vi "ClearTable.vi"(8 "error in":errorcluster, 10 "Table Name":string, 11 "Path":path) -> (0 "error out":errorcluster, 1 "OK？":bool, 2 "Table Name":string, 3 "Path":path)   [LabVIEW 2017, in "SQLite.lvlib"]
uses:
  SQLite.lvlib
  Core/Tables/SQLite_Clear Table.vi
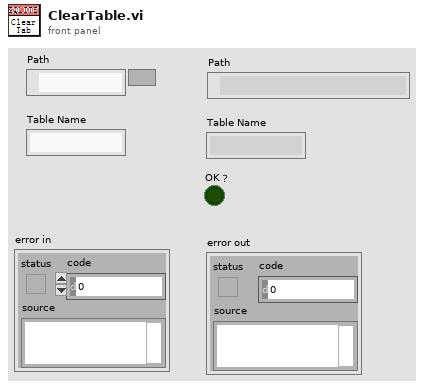
[diagram p1: front panel]
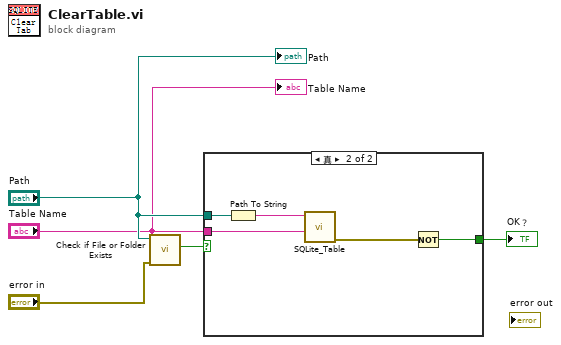
[diagram p0: block diagram]
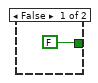
[diagram p2: hidden frame]
diagram:
  n1 = call <vilib>:"Check if File or Folder Exists.vi"("error in (no error)"="error in", "path"="Path") -> ("file or folder exists?"=w4:bool)  [unwired: 7 in, 2 out]
  n2 = case shown="真" w4 {
    tunnel: [FALSE w9] -> w5
    tunnel: "Table Name" -> [_ w8]
    tunnel: "Path" -> [_ w7]
    frame False {
    }
    frame True {
      n3 = Path To String(path=w7) -> (string=w11:string)
      n4 = call-poly "SQLite_Table.vi"("DB Path"=w11, "Table Name"=w8) -> ("error out"=w10:errorcluster)  [unwired: 6 in, 2 out]
      n5 = Not(x=w10) -> (.not. x?=w9:bool)
    }
  }
  "OK？" <- w5
  "Path" <- "Path"
  "Table Name" <- "Table Name"
